vi "Init.vi"(8 "error in (no error)":errorcluster, 10 "Node Reg":refnum<k20>, 11 "MultiDiagramStructure in":refnum<class "MultiDiagramStructure.lvclass">) -> (0 "error out":errorcluster, 3 "MultiDiagramStructure out":refnum<class "MultiDiagramStructure.lvclass">)   [LabVIEW 2025, in "MultiDiagramStructure.lvclass"]
uses:
  MultiDiagramStructure.lvclass
  Controls/Subdiagram.ctl
  Node.lvclass
  MultiDiagramStructure.lvclass/MultiDiagramStructure.ctl
  <vilib>/xml/NI_XML.lvlib
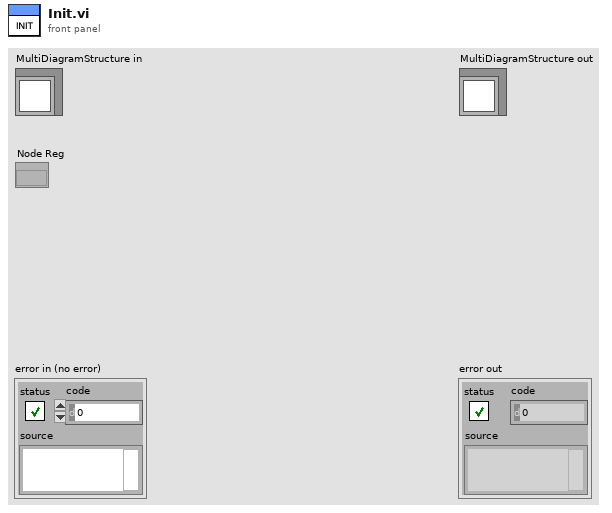
[diagram p1: front panel]
types:
  T1 = typedef "Subdiagram.ctl" = cluster{"diagram":refnum<vi>, "selector":string, "uuid":string}
  T2 = typedef "Tunnel.ctl" = cluster{"OuterUUID":T3, "InnerUUIDs":T3[]}
  T3 = typedef "Terminal.ctl" = cluster{"id":string, "name":string, "terminal":refnum<vi>}
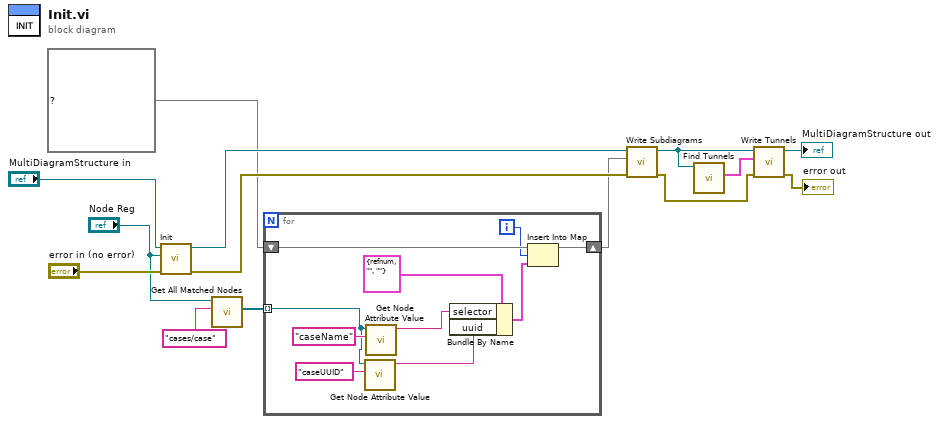
[diagram p0: block diagram]
diagram:
  n1 = call-parent "Init.vi"("error in (no error)"="error in (no error)", "Node Reg"="Node Reg", "Node in"="MultiDiagramStructure in") -> ("error out"=w8:errorcluster, "Node out"=w9:refnum<class "MultiDiagramStructure.lvclass">)  [unwired: 7 in]
  n2 = call <vilib>:"Get All Matched Nodes.vi"("XPath expression"="cases/case", "node in"="Node Reg") -> ("node result array"=w10:refnum<k20>[])  [unwired: 7 in, 2 out]
  n3 = for {
    tunnel: w10 -> [w22] mode=indexing
    shift-right: [w20] -> w6
    shift-left: map{u64, T1} {} ("Subdiagrams") -> [w21]
    i -> [w15]
    n4 = call "Get Node Attribute Value.vi"("Attribute Name"="caseUUID", "Refnum in"=w22) -> ("Value"=w16:string)  [unwired: 9 in]
    n5 = call "Get Node Attribute Value.vi"("Attribute Name"="caseName", "Refnum in"=w22) -> ("Value"=w17:string)  [unwired: 9 in]
    n6 = Bundle By Name(cluster=T1 {"diagram"=refnum, "selector"="", "uuid"=""} ("value"), "selector"=w17, "uuid"=w16) -> (w18:T1)
    n7 = Insert Into Map(map in=w21, key=w15, value=w18) -> (map out=w20:map{u64, T1})  [unwired: 2 out]
  }
  n8 = call-dynamic "Write Subdiagrams.vi"("error in (no error)"=w8, "Subdiagrams"=w6, "MultiDiagramStructure in"=w9) -> ("error out"=w3:errorcluster, "MultiDiagramStructure out"=w5:refnum<class "MultiDiagramStructure.lvclass">)  [unwired: 7 in]
  n9 = call "Find Tunnels.vi"("MultiDiagramStructure in"=w5) -> ("Tunnel Array"=w1:T2[])  [unwired: 9 in, 1 out]
  n10 = call-dynamic "Write Tunnels.vi"("error in (no error)"=w3, "Tunnels"=w1, "MultiDiagramStructure in"=w5) -> ("error out"=→"error out":errorcluster, "MultiDiagramStructure out"=→"MultiDiagramStructure out":refnum<class "MultiDiagramStructure.lvclass">)  [unwired: 7 in]
